vi "RTS Wago Data 1.vi"(8 "Error In":errorcluster, 11 "Chamber 1 Data in":T1 {"Room PID Settings"."Room Dehumid Temperature I (*RM Dehum I1)" max=30000 step=1; "Room PID Settings"."Room Dehumid Temperature P (*RM Dehum P1)" max=30000 step=1; "Room PID Settings"."Room Cool Temperature I (*RM Cool I1)" max=30000 step=1; "Room PID Settings"."Room Cool Temperature P (*RM Cool P1)" max=30000 step=1; "Room PID Settings"."Room Heat I (*RM Heat I1)" max=30000 step=1; "Room PID Settings"."Room Heat P (*RM Heat P1)" max=30000 step=1; "Room PID Settings"."Room Humidity I (*RM Hum I1)" max=30000 step=1; "Room PID Settings"."Room Humidity P (*RM Hum P1)" max=30000 step=1; "Room PID Settings"."Room Dry I (*RM Dry I1)" max=30000 step=1; "Room PID Settings"."Room Dry P(*RM Dry P1)" max=30000 step=1; "Station 8"."Voltage (V):Element 1 Avg" format="%.3g"; "Station 8"."Voltage (V):Element 2 Avg" format="%.3g"; "Station 8"."Max Watt Hours" format="%.3g"; "Station 8"."Power Factor:Element 2" format="%.3g"; "Station 8"."Power Factor:Element 1" format="%.3g"; "Station 8"."Apparent Power (VA):Element 2" format="%.3g"; "Station 8"."Apparent Power (VA):Element 1" format="%.3g"; "Station 8"."Frequency (Hz):Element 1" format="%.3g"; "Station 8"."Time:Element 1" format="%.3g"; "Station 8"."Voltage Crest Factor:Element 2" format="%.3g"; "Station 8"."Voltage Crest Factor:Element 1" format="%.3g"; "Station 8"."Voltage Harmonic (%):Element 2" format="%.3g"; "Station 8"."Voltage Harmonic (%):Element 1" format="%.3g"; "Station 8"."Current Crest Factor:Element 2" format="%.3g"; "Station 8"."Current Crest Factor:Element 1" format="%.3g"; "Station 8"."Voltage (V):Element 1" format="%.3g"; "Station 8"."Voltage (V):Element 2" format="%.3g"; "Station 8"."Watt Hours (Wh):Sigma" format="%.3f"; "Station 8"."Power (W):Sigma" format="%.3g"; "Station 8"."Current (A):Element 2" format="%.3g"; "Station 8"."Current (A):Element 1" format="%.3g"; "Station 7"."Voltage (V):Element 1 Avg" format="%.3g"; "Station 7"."Voltage (V):Element 2 Avg" format="%.3g"; "Station 7"."Max Watt Hours" format="%.3g"; "Station 7"."Power Factor:Element 2" format="%.3g"; "Station 7"."Power Factor:Element 1" format="%.3g"; "Station 7"."Apparent Power (VA):Element 2" format="%.3g"; "Station 7"."Apparent Power (VA):Element 1" format="%.3g"; "Station 7"."Frequency (Hz):Element 1" format="%.3g"; "Station 7"."Time:Element 1" format="%.3g"; "Station 7"."Voltage Crest Factor:Element 2" format="%.3g"; "Station 7"."Voltage Crest Factor:Element 1" format="%.3g"; "Station 7"."Voltage Harmonic (%):Element 2" format="%.3g"; "Station 7"."Voltage Harmonic (%):Element 1" format="%.3g"; "Station 7"."Current Crest Factor:Element 2" format="%.3g"; "Station 7"."Current Crest Factor:Element 1" format="%.3g"; "Station 7"."Voltage (V):Element 1" format="%.3g"; "Station 7"."Voltage (V):Element 2" format="%.3g"; "Station 7"."Watt Hours (Wh):Sigma" format="%.3f"; "Station 7"."Power (W):Sigma" format="%.3g"; "Station 7"."Current (A):Element 2" format="%.3g"; "Station 7"."Current (A):Element 1" format="%.3g"; "Station 6"."Voltage (V):Element 1 Avg" format="%.3g"; "Station 6"."Voltage (V):Element 2 Avg" format="%.3g"; "Station 6"."Max Watt Hours" format="%.3g"; "Station 6"."Power Factor:Element 2" format="%.3g"; "Station 6"."Power Factor:Element 1" format="%.3g"; "Station 6"."Apparent Power (VA):Element 2" format="%.3g"; "Station 6"."Apparent Power (VA):Element 1" format="%.3g"; "Station 6"."Frequency (Hz):Element 1" format="%.3g"; "Station 6"."Time:Element 1" format="%.3g"; "Station 6"."Voltage Crest Factor:Element 2" format="%.3g"; "Station 6"."Voltage Crest Factor:Element 1" format="%.3g"; "Station 6"."Voltage Harmonic (%):Element 2" format="%.3g"; "Station 6"."Voltage Harmonic (%):Element 1" format="%.3g"; "Station 6"."Current Crest Factor:Element 2" format="%.3g"; "Station 6"."Current Crest Factor:Element 1" format="%.3g"; "Station 6"."Voltage (V):Element 1" format="%.3g"; "Station 6"."Voltage (V):Element 2" format="%.3g"; "Station 6"."Watt Hours (Wh):Sigma" format="%.3f"; "Station 6"."Power (W):Sigma" format="%.3g"; "Station 6"."Current (A):Element 2" format="%.3g"; "Station 6"."Current (A):Element 1" format="%.3g"; "Station 5"."Voltage (V):Element 1 Avg" format="%.3g"; "Station 5"."Voltage (V):Element 2 Avg" format="%.3g"; "Station 5"."Max Watt Hours" format="%.3g"; "Station 5"."Power Factor:Element 2" format="%.3g"; "Station 5"."Power Factor:Element 1" format="%.3g"; "Station 5"."Apparent Power (VA):Element 2" format="%.3g"; "Station 5"."Apparent Power (VA):Element 1" format="%.3g"; "Station 5"."Frequency (Hz):Element 1" format="%.3g"; "Station 5"."Time:Element 1" format="%.3g"; "Station 5"."Voltage Crest Factor:Element 2" format="%.3g"; "Station 5"."Voltage Crest Factor:Element 1" format="%.3g"; "Station 5"."Voltage Harmonic (%):Element 2" format="%.3g"; "Station 5"."Voltage Harmonic (%):Element 1" format="%.3g"; "Station 5"."Current Crest Factor:Element 2" format="%.3g"; "Station 5"."Current Crest Factor:Element 1" format="%.3g"; "Station 5"."Voltage (V):Element 1" format="%.3g"; "Station 5"."Voltage (V):Element 2" format="%.3g"; "Station 5"."Watt Hours (Wh):Sigma" format="%.3f"; "Station 5"."Power (W):Sigma" format="%.3g"; "Station 5"."Current (A):Element 2" format="%.3g"; "Station 5"."Current (A):Element 1" format="%.3g"; "Station 4"."Voltage (V):Element 1 Avg" format="%.3g"; "Station 4"."Voltage (V):Element 2 Avg" format="%.3g"; "Station 4"."Max Watt Hours" format="%.3g"; "Station 4"."Power Factor:Element 2" format="%.3g"; "Station 4"."Power Factor:Element 1" format="%.3g"; "Station 4"."Apparent Power (VA):Element 2" format="%.3g"; "Station 4"."Apparent Power (VA):Element 1" format="%.3g"; "Station 4"."Frequency (Hz):Element 1" format="%.3g"; "Station 4"."Time:Element 1" format="%.3g"; "Station 4"."Voltage Crest Factor:Element 2" format="%.3g"; "Station 4"."Voltage Crest Factor:Element 1" format="%.3g"; "Station 4"."Voltage Harmonic (%):Element 2" format="%.3g"; "Station 4"."Voltage Harmonic (%):Element 1" format="%.3g"; "Station 4"."Current Crest Factor:Element 2" format="%.3g"; "Station 4"."Current Crest Factor:Element 1" format="%.3g"; "Station 4"."Voltage (V):Element 1" format="%.3g"; "Station 4"."Voltage (V):Element 2" format="%.3g"; "Station 4"."Watt Hours (Wh):Sigma" format="%.3f"; "Station 4"."Power (W):Sigma" format="%.3g"; "Station 4"."Current (A):Element 2" format="%.3g"; "Station 4"."Current (A):Element 1" format="%.3g"; "Station 3"."Voltage (V):Element 1 Avg" format="%.3g"; "Station 3"."Voltage (V):Element 2 Avg" format="%.3g"; "Station 3"."Max Watt Hours" format="%.3g"; "Station 3"."Power Factor:Element 2" format="%.3g"; "Station 3"."Power Factor:Element 1" format="%.3g"; "Station 3"."Apparent Power (VA):Element 2" format="%.3g"; "Station 3"."Apparent Power (VA):Element 1" format="%.3g"; "Station 3"."Frequency (Hz):Element 1" format="%.3g"; "Station 3"."Time:Element 1" format="%.3g"; "Station 3"."Voltage Crest Factor:Element 2" format="%.3g"; "Station 3"."Voltage Crest Factor:Element 1" format="%.3g"; "Station 3"."Voltage Harmonic (%):Element 2" format="%.3g"; "Station 3"."Voltage Harmonic (%):Element 1" format="%.3g"; "Station 3"."Current Crest Factor:Element 2" format="%.3g"; "Station 3"."Current Crest Factor:Element 1" format="%.3g"; "Station 3"."Voltage (V):Element 1" format="%.3g"; "Station 3"."Voltage (V):Element 2" format="%.3g"; "Station 3"."Watt Hours (Wh):Sigma" format="%.3f"; "Station 3"."Power (W):Sigma" format="%.3g"; "Station 3"."Current (A):Element 2" format="%.3g"; "Station 3"."Current (A):Element 1" format="%.3g"; "Station 2"."Voltage (V):Element 1 Avg" format="%.3g"; "Station 2"."Voltage (V):Element 2 Avg" format="%.3g"; "Station 2"."Max Watt Hours" format="%.3g"; "Station 2"."Power Factor:Element 2" format="%.3g"; "Station 2"."Power Factor:Element 1" format="%.3g"; "Station 2"."Apparent Power (VA):Element 2" format="%.3g"; "Station 2"."Apparent Power (VA):Element 1" format="%.3g"; "Station 2"."Frequency (Hz):Element 1" format="%.3g"; "Station 2"."Time:Element 1" format="%.3g"; "Station 2"."Voltage Crest Factor:Element 2" format="%.3g"; "Station 2"."Voltage Crest Factor:Element 1" format="%.3g"; "Station 2"."Voltage Harmonic (%):Element 2" format="%.3g"; "Station 2"."Voltage Harmonic (%):Element 1" format="%.3g"; "Station 2"."Current Crest Factor:Element 2" format="%.3g"; "Station 2"."Current Crest Factor:Element 1" format="%.3g"; "Station 2"."Voltage (V):Element 1" format="%.3g"; "Station 2"."Voltage (V):Element 2" format="%.3g"; "Station 2"."Watt Hours (Wh):Sigma" format="%.3f"; "Station 2"."Power (W):Sigma" format="%.3g"; "Station 2"."Current (A):Element 2" format="%.3g"; "Station 2"."Current (A):Element 1" format="%.3g"; "Station 1"."Voltage (V):Element 1 Avg" format="%.3g"; "Station 1"."Voltage (V):Element 2 Avg" format="%.3g"; "Station 1"."Max Watt Hours" format="%.3g"; "Station 1"."Power Factor:Element 2" format="%.3g"; "Station 1"."Power Factor:Element 1" format="%.3g"; "Station 1"."Apparent Power (VA):Element 2" format="%.3g"; "Station 1"."Apparent Power (VA):Element 1" format="%.3g"; "Station 1"."Frequency (Hz):Element 1" format="%.3g"; "Station 1"."Time:Element 1" format="%.3g"; "Station 1"."Voltage Crest Factor:Element 2" format="%.3g"; "Station 1"."Voltage Crest Factor:Element 1" format="%.3g"; "Station 1"."Voltage Harmonic (%):Element 2" format="%.3g"; "Station 1"."Voltage Harmonic (%):Element 1" format="%.3g"; "Station 1"."Current Crest Factor:Element 2" format="%.3g"; "Station 1"."Current Crest Factor:Element 1" format="%.3g"; "Station 1"."Voltage (V):Element 1" format="%.3g"; "Station 1"."Voltage (V):Element 2" format="%.3g"; "Station 1"."Watt Hours (Wh):Sigma" format="%.3f"; "Station 1"."Power (W):Sigma" format="%.3g"; "Station 1"."Current (A):Element 2" format="%.3g"; "Station 1"."Current (A):Element 1" format="%.3g"}) -> (0 "Error Out":errorcluster, 1 "Data (DBL)":dbl[](array[numeric]), 2 "Data 1 Output":string[][](array[string]), 3 "Chamber 1 Data Out":T1 {"Room PID Settings"."Room Dehumid Temperature I (*RM Dehum I1)" max=30000 step=1; "Room PID Settings"."Room Dehumid Temperature P (*RM Dehum P1)" max=30000 step=1; "Room PID Settings"."Room Cool Temperature I (*RM Cool I1)" max=30000 step=1; "Room PID Settings"."Room Cool Temperature P (*RM Cool P1)" max=30000 step=1; "Room PID Settings"."Room Heat I (*RM Heat I1)" max=30000 step=1; "Room PID Settings"."Room Heat P (*RM Heat P1)" max=30000 step=1; "Room PID Settings"."Room Humidity I (*RM Hum I1)" max=30000 step=1; "Room PID Settings"."Room Humidity P (*RM Hum P1)" max=30000 step=1; "Room PID Settings"."Room Dry I (*RM Dry I1)" max=30000 step=1; "Room PID Settings"."Room Dry P(*RM Dry P1)" max=30000 step=1; "Station 8"."Voltage (V):Element 1 Avg" format="%.3g"; "Station 8"."Voltage (V):Element 2 Avg" format="%.3g"; "Station 8"."Max Watt Hours" format="%.3g"; "Station 8"."Power Factor:Element 2" format="%.3g"; "Station 8"."Power Factor:Element 1" format="%.3g"; "Station 8"."Apparent Power (VA):Element 2" format="%.3g"; "Station 8"."Apparent Power (VA):Element 1" format="%.3g"; "Station 8"."Frequency (Hz):Element 1" format="%.3g"; "Station 8"."Time:Element 1" format="%.3g"; "Station 8"."Voltage Crest Factor:Element 2" format="%.3g"; "Station 8"."Voltage Crest Factor:Element 1" format="%.3g"; "Station 8"."Voltage Harmonic (%):Element 2" format="%.3g"; "Station 8"."Voltage Harmonic (%):Element 1" format="%.3g"; "Station 8"."Current Crest Factor:Element 2" format="%.3g"; "Station 8"."Current Crest Factor:Element 1" format="%.3g"; "Station 8"."Voltage (V):Element 1" format="%.3g"; "Station 8"."Voltage (V):Element 2" format="%.3g"; "Station 8"."Watt Hours (Wh):Sigma" format="%.3f"; "Station 8"."Power (W):Sigma" format="%.3g"; "Station 8"."Current (A):Element 2" format="%.3g"; "Station 8"."Current (A):Element 1" format="%.3g"; "Station 7"."Voltage (V):Element 1 Avg" format="%.3g"; "Station 7"."Voltage (V):Element 2 Avg" format="%.3g"; "Station 7"."Max Watt Hours" format="%.3g"; "Station 7"."Power Factor:Element 2" format="%.3g"; "Station 7"."Power Factor:Element 1" format="%.3g"; "Station 7"."Apparent Power (VA):Element 2" format="%.3g"; "Station 7"."Apparent Power (VA):Element 1" format="%.3g"; "Station 7"."Frequency (Hz):Element 1" format="%.3g"; "Station 7"."Time:Element 1" format="%.3g"; "Station 7"."Voltage Crest Factor:Element 2" format="%.3g"; "Station 7"."Voltage Crest Factor:Element 1" format="%.3g"; "Station 7"."Voltage Harmonic (%):Element 2" format="%.3g"; "Station 7"."Voltage Harmonic (%):Element 1" format="%.3g"; "Station 7"."Current Crest Factor:Element 2" format="%.3g"; "Station 7"."Current Crest Factor:Element 1" format="%.3g"; "Station 7"."Voltage (V):Element 1" format="%.3g"; "Station 7"."Voltage (V):Element 2" format="%.3g"; "Station 7"."Watt Hours (Wh):Sigma" format="%.3f"; "Station 7"."Power (W):Sigma" format="%.3g"; "Station 7"."Current (A):Element 2" format="%.3g"; "Station 7"."Current (A):Element 1" format="%.3g"; "Station 6"."Voltage (V):Element 1 Avg" format="%.3g"; "Station 6"."Voltage (V):Element 2 Avg" format="%.3g"; "Station 6"."Max Watt Hours" format="%.3g"; "Station 6"."Power Factor:Element 2" format="%.3g"; "Station 6"."Power Factor:Element 1" format="%.3g"; "Station 6"."Apparent Power (VA):Element 2" format="%.3g"; "Station 6"."Apparent Power (VA):Element 1" format="%.3g"; "Station 6"."Frequency (Hz):Element 1" format="%.3g"; "Station 6"."Time:Element 1" format="%.3g"; "Station 6"."Voltage Crest Factor:Element 2" format="%.3g"; "Station 6"."Voltage Crest Factor:Element 1" format="%.3g"; "Station 6"."Voltage Harmonic (%):Element 2" format="%.3g"; "Station 6"."Voltage Harmonic (%):Element 1" format="%.3g"; "Station 6"."Current Crest Factor:Element 2" format="%.3g"; "Station 6"."Current Crest Factor:Element 1" format="%.3g"; "Station 6"."Voltage (V):Element 1" format="%.3g"; "Station 6"."Voltage (V):Element 2" format="%.3g"; "Station 6"."Watt Hours (Wh):Sigma" format="%.3f"; "Station 6"."Power (W):Sigma" format="%.3g"; "Station 6"."Current (A):Element 2" format="%.3g"; "Station 6"."Current (A):Element 1" format="%.3g"; "Station 5"."Voltage (V):Element 1 Avg" format="%.3g"; "Station 5"."Voltage (V):Element 2 Avg" format="%.3g"; "Station 5"."Max Watt Hours" format="%.3g"; "Station 5"."Power Factor:Element 2" format="%.3g"; "Station 5"."Power Factor:Element 1" format="%.3g"; "Station 5"."Apparent Power (VA):Element 2" format="%.3g"; "Station 5"."Apparent Power (VA):Element 1" format="%.3g"; "Station 5"."Frequency (Hz):Element 1" format="%.3g"; "Station 5"."Time:Element 1" format="%.3g"; "Station 5"."Voltage Crest Factor:Element 2" format="%.3g"; "Station 5"."Voltage Crest Factor:Element 1" format="%.3g"; "Station 5"."Voltage Harmonic (%):Element 2" format="%.3g"; "Station 5"."Voltage Harmonic (%):Element 1" format="%.3g"; "Station 5"."Current Crest Factor:Element 2" format="%.3g"; "Station 5"."Current Crest Factor:Element 1" format="%.3g"; "Station 5"."Voltage (V):Element 1" format="%.3g"; "Station 5"."Voltage (V):Element 2" format="%.3g"; "Station 5"."Watt Hours (Wh):Sigma" format="%.3f"; "Station 5"."Power (W):Sigma" format="%.3g"; "Station 5"."Current (A):Element 2" format="%.3g"; "Station 5"."Current (A):Element 1" format="%.3g"; "Station 4"."Voltage (V):Element 1 Avg" format="%.3g"; "Station 4"."Voltage (V):Element 2 Avg" format="%.3g"; "Station 4"."Max Watt Hours" format="%.3g"; "Station 4"."Power Factor:Element 2" format="%.3g"; "Station 4"."Power Factor:Element 1" format="%.3g"; "Station 4"."Apparent Power (VA):Element 2" format="%.3g"; "Station 4"."Apparent Power (VA):Element 1" format="%.3g"; "Station 4"."Frequency (Hz):Element 1" format="%.3g"; "Station 4"."Time:Element 1" format="%.3g"; "Station 4"."Voltage Crest Factor:Element 2" format="%.3g"; "Station 4"."Voltage Crest Factor:Element 1" format="%.3g"; "Station 4"."Voltage Harmonic (%):Element 2" format="%.3g"; "Station 4"."Voltage Harmonic (%):Element 1" format="%.3g"; "Station 4"."Current Crest Factor:Element 2" format="%.3g"; "Station 4"."Current Crest Factor:Element 1" format="%.3g"; "Station 4"."Voltage (V):Element 1" format="%.3g"; "Station 4"."Voltage (V):Element 2" format="%.3g"; "Station 4"."Watt Hours (Wh):Sigma" format="%.3f"; "Station 4"."Power (W):Sigma" format="%.3g"; "Station 4"."Current (A):Element 2" format="%.3g"; "Station 4"."Current (A):Element 1" format="%.3g"; "Station 3"."Voltage (V):Element 1 Avg" format="%.3g"; "Station 3"."Voltage (V):Element 2 Avg" format="%.3g"; "Station 3"."Max Watt Hours" format="%.3g"; "Station 3"."Power Factor:Element 2" format="%.3g"; "Station 3"."Power Factor:Element 1" format="%.3g"; "Station 3"."Apparent Power (VA):Element 2" format="%.3g"; "Station 3"."Apparent Power (VA):Element 1" format="%.3g"; "Station 3"."Frequency (Hz):Element 1" format="%.3g"; "Station 3"."Time:Element 1" format="%.3g"; "Station 3"."Voltage Crest Factor:Element 2" format="%.3g"; "Station 3"."Voltage Crest Factor:Element 1" format="%.3g"; "Station 3"."Voltage Harmonic (%):Element 2" format="%.3g"; "Station 3"."Voltage Harmonic (%):Element 1" format="%.3g"; "Station 3"."Current Crest Factor:Element 2" format="%.3g"; "Station 3"."Current Crest Factor:Element 1" format="%.3g"; "Station 3"."Voltage (V):Element 1" format="%.3g"; "Station 3"."Voltage (V):Element 2" format="%.3g"; "Station 3"."Watt Hours (Wh):Sigma" format="%.3f"; "Station 3"."Power (W):Sigma" format="%.3g"; "Station 3"."Current (A):Element 2" format="%.3g"; "Station 3"."Current (A):Element 1" format="%.3g"; "Station 2"."Voltage (V):Element 1 Avg" format="%.3g"; "Station 2"."Voltage (V):Element 2 Avg" format="%.3g"; "Station 2"."Max Watt Hours" format="%.3g"; "Station 2"."Power Factor:Element 2" format="%.3g"; "Station 2"."Power Factor:Element 1" format="%.3g"; "Station 2"."Apparent Power (VA):Element 2" format="%.3g"; "Station 2"."Apparent Power (VA):Element 1" format="%.3g"; "Station 2"."Frequency (Hz):Element 1" format="%.3g"; "Station 2"."Time:Element 1" format="%.3g"; "Station 2"."Voltage Crest Factor:Element 2" format="%.3g"; "Station 2"."Voltage Crest Factor:Element 1" format="%.3g"; "Station 2"."Voltage Harmonic (%):Element 2" format="%.3g"; "Station 2"."Voltage Harmonic (%):Element 1" format="%.3g"; "Station 2"."Current Crest Factor:Element 2" format="%.3g"; "Station 2"."Current Crest Factor:Element 1" format="%.3g"; "Station 2"."Voltage (V):Element 1" format="%.3g"; "Station 2"."Voltage (V):Element 2" format="%.3g"; "Station 2"."Watt Hours (Wh):Sigma" format="%.3f"; "Station 2"."Power (W):Sigma" format="%.3g"; "Station 2"."Current (A):Element 2" format="%.3g"; "Station 2"."Current (A):Element 1" format="%.3g"; "Station 1"."Voltage (V):Element 1 Avg" format="%.3g"; "Station 1"."Voltage (V):Element 2 Avg" format="%.3g"; "Station 1"."Max Watt Hours" format="%.3g"; "Station 1"."Power Factor:Element 2" format="%.3g"; "Station 1"."Power Factor:Element 1" format="%.3g"; "Station 1"."Apparent Power (VA):Element 2" format="%.3g"; "Station 1"."Apparent Power (VA):Element 1" format="%.3g"; "Station 1"."Frequency (Hz):Element 1" format="%.3g"; "Station 1"."Time:Element 1" format="%.3g"; "Station 1"."Voltage Crest Factor:Element 2" format="%.3g"; "Station 1"."Voltage Crest Factor:Element 1" format="%.3g"; "Station 1"."Voltage Harmonic (%):Element 2" format="%.3g"; "Station 1"."Voltage Harmonic (%):Element 1" format="%.3g"; "Station 1"."Current Crest Factor:Element 2" format="%.3g"; "Station 1"."Current Crest Factor:Element 1" format="%.3g"; "Station 1"."Voltage (V):Element 1" format="%.3g"; "Station 1"."Voltage (V):Element 2" format="%.3g"; "Station 1"."Watt Hours (Wh):Sigma" format="%.3f"; "Station 1"."Power (W):Sigma" format="%.3g"; "Station 1"."Current (A):Element 2" format="%.3g"; "Station 1"."Current (A):Element 1" format="%.3g"})   [LabVIEW 2016]
uses:
  Type Definitions/RTS Chamber Data.ctl
  Utility/Type Definitions/UTILITY Power Data.ctl
  Type Definitions/RTS Chamber TCs.ctl
  Type Definitions/RTS MX5 AUX Data.ctl
  Drivers/WAGO 750-881/Type Definitions/Wago Door Relays.ctl
  Drivers/WAGO 750-881/Type Definitions/Wago Contactor Settings.ctl
  Drivers/WAGO 750-881/Type Definitions/Wago Ground Leakage.ctl
  Drivers/WAGO 750-881/Type Definitions/Wago Measured Input Data.ctl
  Drivers/WAGO 750-881/Type Definitions/Wago Room Setpoint Targets.ctl
  Drivers/WAGO 750-881/Type Definitions/Wago Room PID Settings.ctl
  Drivers/WAGO 750-881/Type Definitions/Wago Room Condtions.ctl
panel:
  # "APLUS"
  # "MX100"
  # "Wago Controller"
  # "APLUS"
  # "MX100"
  # "Wago Controller"
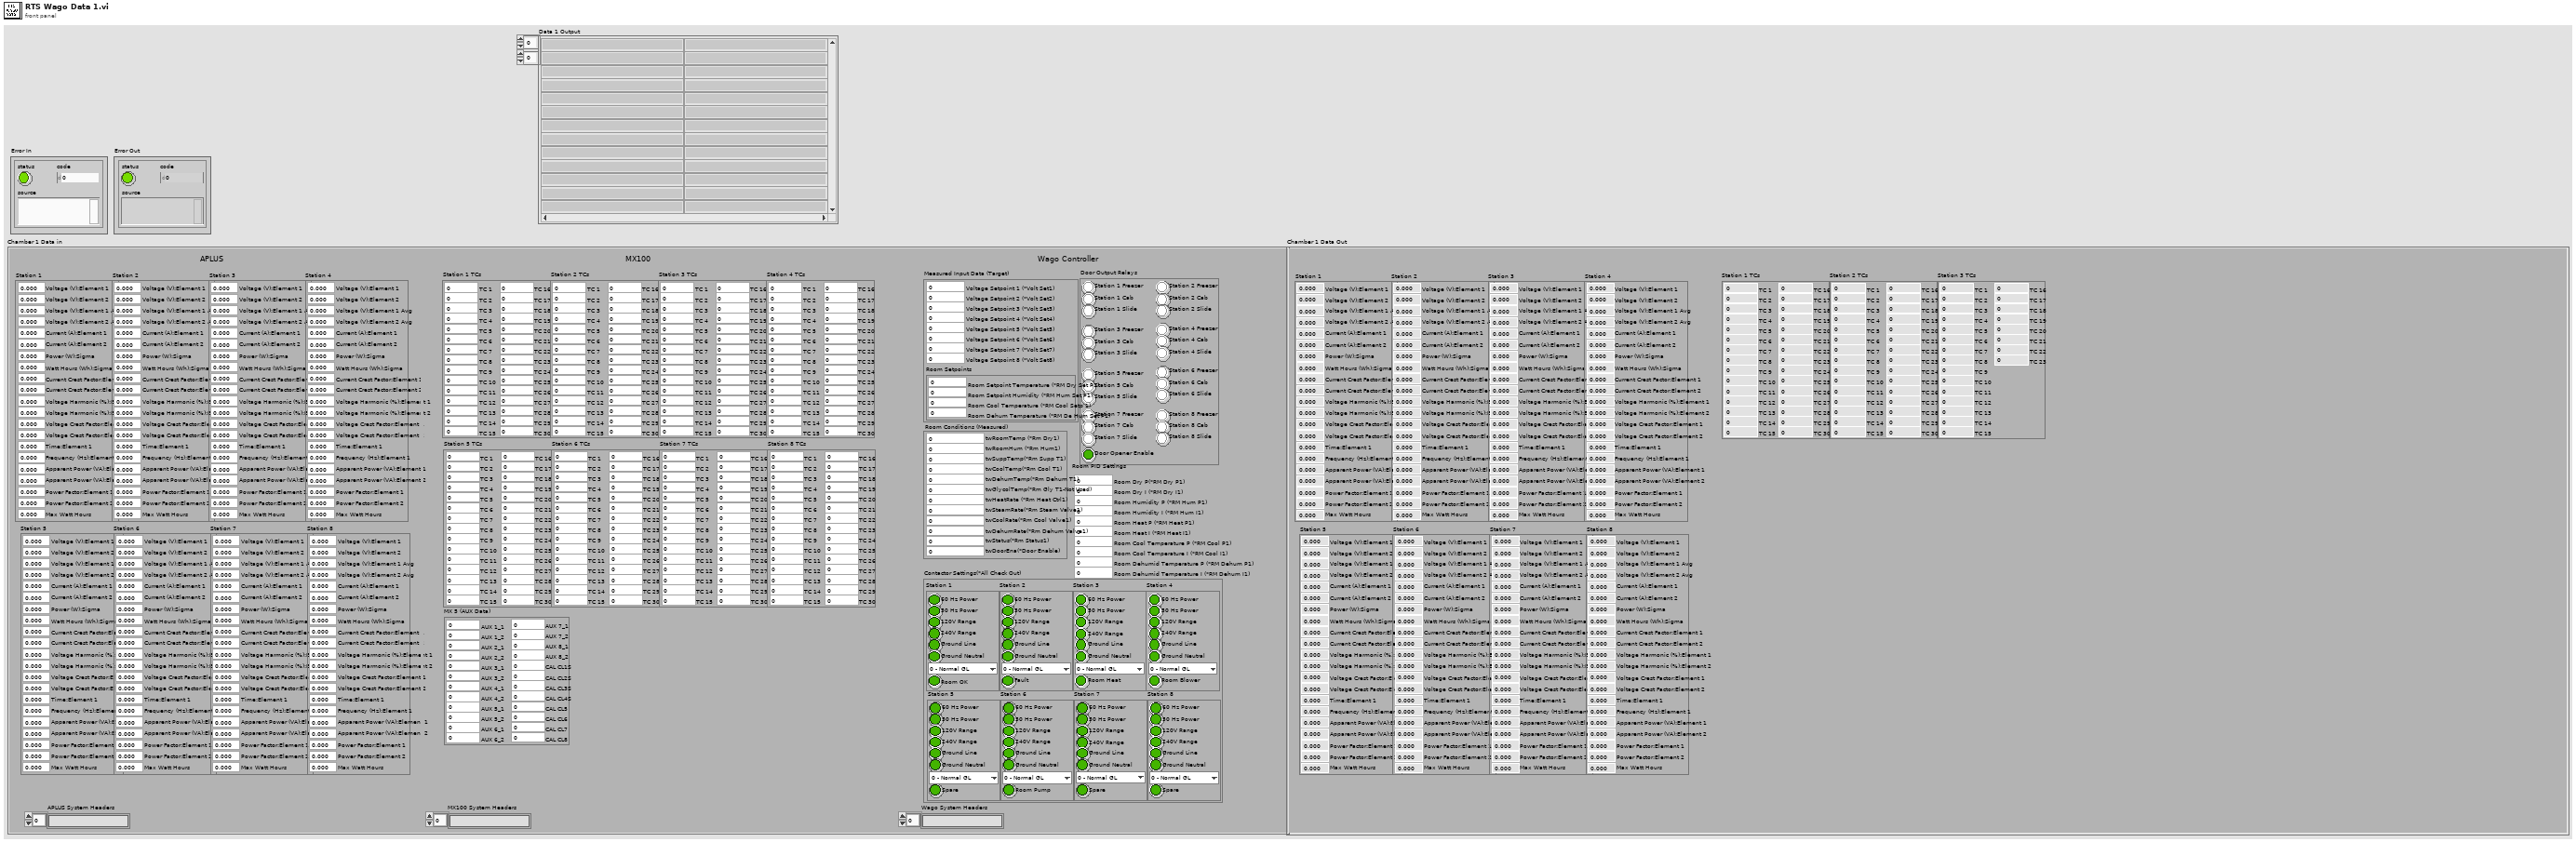
[diagram p1: front panel]
types:
  T1 = typedef "RTS Chamber Data.ctl" = cluster{"Station 1":T2, "Station 2":T2, "Station 3":T2, "Station 4":T2, "Station 5":T2, "Station 6":T2, "Station 7":T2, "Station 8":T2, "Station 1 TCs":T3, "Station 2 TCs":T3, "Station 3 TCs":T3, "Station 4 TCs":T3, "Station 5 TCs":T3, "Station 6 TCs":T3, "Station 7 TCs":T3, "Station 8 TCs":T3, "MX 5 (AUX Data)":T4, "Door Output Relays":T5, "Contactor Settings(*All Check Out)":T6, "Measured Input Data (Target)":T8, "Room PID Settings":T10, "Room Conditions (Measured)":T11, "APLUS System Headers":string[], "MX100 System Headers":string[], "Wago System Headers":string[]}
  T2 = typedef "UTILITY Power Data.ctl" = cluster{"Current (A):Element 1":dbl, "Current (A):Element 2":dbl, "Power (W):Sigma":dbl, "Watt Hours (Wh):Sigma":dbl, "Voltage (V):Element 2":dbl, "Voltage (V):Element 1":dbl, "Current Crest Factor:Element 1":dbl, "Current Crest Factor:Element 2":dbl, "Voltage Harmonic (%):Element 1":dbl, "Voltage Harmonic (%):Element 2":dbl, "Voltage Crest Factor:Element 1":dbl, "Voltage Crest Factor:Element 2":dbl, "Time:Element 1":dbl, "Frequency (Hz):Element 1":dbl, "Apparent Power (VA):Element 1":dbl, "Apparent Power (VA):Element 2":dbl, "Power Factor:Element 1":dbl, "Power Factor:Element 2":dbl, "Max Watt Hours":dbl, "Voltage (V):Element 2 Avg":dbl, "Voltage (V):Element 1 Avg":dbl}
  T3 = typedef "RTS Chamber TCs.ctl" = cluster{"TC 1":dbl, "TC 2":dbl, "TC 3":dbl, "TC 4":dbl, "TC 5":dbl, "TC 6":dbl, "TC 7":dbl, "TC 8":dbl, "TC 9":dbl, "TC 10":dbl, "TC 11":dbl, "TC 12":dbl, "TC 13":dbl, "TC 14":dbl, "TC 15":dbl, "TC 16":dbl, "TC 17":dbl, "TC 18":dbl, "TC 19":dbl, "TC 20":dbl, "TC 21":dbl, "TC 22":dbl, "TC 23":dbl, "TC 24":dbl, "TC 25":dbl, "TC 26":dbl, "TC 27":dbl, "TC 28":dbl, "TC 29":dbl, "TC 30":dbl}
  T4 = typedef "RTS MX5 AUX Data.ctl" = cluster{"AUX 1_1":dbl, "AUX 1_2":dbl, "AUX 2_1":dbl, "AUX 2_2":dbl, "AUX 3_1":dbl, "AUX 3_2":dbl, "AUX 4_1":dbl, "AUX 4_2":dbl, "AUX 5_1":dbl, "AUX 5_2":dbl, "AUX 6_1":dbl, "AUX 6_2":dbl, "AUX 7_1":dbl, "AUX 7_2":dbl, "AUX 8_1":dbl, "AUX 8_2":dbl, "CAL CL1S":dbl, "CAL CL2S":dbl, "CAL CL3S":dbl, "CAL CL4S":dbl, "CAL CL5":dbl, "CAL CL6":dbl, "CAL CL7":dbl, "CAL CL8":dbl}
  T5 = typedef "Wago Door Relays.ctl" = cluster{"Station 1 Freezer":bool, "Station 1 Cab":bool, "Station 1 Slide":bool, "Station 2 Freezer":bool, "Station 2 Cab":bool, "Station 2 Slide":bool, "Station 3 Freezer":bool, "Station 3 Cab":bool, "Station 3 Slide":bool, "Station 4 Freezer":bool, "Station 4 Cab":bool, "Station 4 Slide":bool, "Station 5 Freezer":bool, "Station 5 Cab":bool, "Station 5 Slide":bool, "Station 6 Freezer":bool, "Station 6 Cab":bool, "Station 6 Slide":bool, "Station 7 Freezer":bool, "Station 7 Cab":bool, "Station 7 Slide":bool, "Station 8 Freezer":bool, "Station 8 Cab":bool, "Station 8 Slide":bool, "Door Opener Enable":bool}
  T6 = typedef "Wago Contactor Settings.ctl" = cluster{"Station 1":cluster{"60 Hz Power":bool, "50 Hz Power":bool, "120V Range":bool, "240V Range":bool, "Ground Line":bool, "Ground Neutral":bool, "Room OK":bool, "Ground Leakage":T7}, "Station 2":cluster{"60 Hz Power":bool, "50 Hz Power":bool, "120V Range":bool, "240V Range":bool, "Ground Line":bool, "Ground Neutral":bool, "Fault":bool, "Ground Leakage":T7}, "Station 3":cluster{"60 Hz Power":bool, "50 Hz Power":bool, "120V Range":bool, "240V Range":bool, "Ground Line":bool, "Ground Neutral":bool, "Room Heat":bool, "Ground Leakage":T7}, "Station 4":cluster{"60 Hz Power":bool, "50 Hz Power":bool, "120V Range":bool, "240V Range":bool, "Ground Line":bool, "Ground Neutral":bool, "Room Blower":bool, "Ground Leakage":T7}, "Station 5":cluster{"60 Hz Power":bool, "50 Hz Power":bool, "120V Range":bool, "240V Range":bool, "Ground Line":bool, "Ground Neutral":bool, "Spare":bool, "Ground Leakage":T7}, "Station 6":cluster{"60 Hz Power":bool, "50 Hz Power":bool, "120V Range":bool, "240V Range":bool, "Ground Line":bool, "Ground Neutral":bool, "Room Pump":bool, "Ground Leakage":T7}, "Station 7":cluster{"60 Hz Power":bool, "50 Hz Power":bool, "120V Range":bool, "240V Range":bool, "Ground Line":bool, "Ground Neutral":bool, "Spare":bool, "Ground Leakage":T7}, "Station 8":cluster{"60 Hz Power":bool, "50 Hz Power":bool, "120V Range":bool, "240V Range":bool, "Ground Line":bool, "Ground Neutral":bool, "Spare":bool, "Ground Leakage":T7}}
  T7 = typedef "Wago Ground Leakage.ctl" = enum16{"0 - Normal GL", "1 - Measure GL"}
  T8 = typedef "Wago Measured Input Data.ctl" = cluster{"Voltage Setpoint 1 (*Volt Set1)":dbl, "Voltage Setpoint 2 (*Volt Set2)":dbl, "Voltage Setpoint 3 (*Volt Set3)":dbl, "Voltage Setpoint 4 (*Volt Set4)":dbl, "Voltage Setpoint 5 (*Volt Set5)":dbl, "Voltage Setpoint 6 (*Volt Set6)":dbl, "Voltage Setpoint 7 (*Volt Set7)":dbl, "Voltage Setpoint 8 (*Volt Set8)":dbl, "Room Setpoints":T9}
  T9 = typedef "Wago Room Setpoint Targets.ctl" = cluster{"Room Setpoint Temperature (*RM Dry Set P1)":dbl, "Room Setpoint Humidity (*RM Hum Set P1)":dbl, "Room Cool Temperature (*RM Cool Setp 1)":dbl, "Room Dehum Temperature (*RM De Hum Set P1)":dbl}
  T10 = typedef "Wago Room PID Settings.ctl" = cluster{"Room Dry P(*RM Dry P1)":u16, "Room Dry I (*RM Dry I1)":u16, "Room Humidity P (*RM Hum P1)":u16, "Room Humidity I (*RM Hum I1)":u16, "Room Heat P (*RM Heat P1)":u16, "Room Heat I (*RM Heat I1)":u16, "Room Cool Temperature P (*RM Cool P1)":u16, "Room Cool Temperature I (*RM Cool I1)":u16, "Room Dehumid Temperature P (*RM Dehum P1)":u16, "Room Dehumid Temperature I (*RM Dehum I1)":u16}
  T11 = typedef "Wago Room Condtions.ctl" = cluster{"twDoorEna(*Door Enable)":u16, "twStatus(*Rm Status1)":u16, "twRoomTemp (*Rm Dry1)":dbl, "twRoomHum (*Rm Hum1)":dbl, "twSuppTemp(*Rm Supp T1)":dbl, "twCoolTemp(*Rm Cool T1)":dbl, "twDehumTemp(*Rm Dehum T1)":dbl, "twGlycolTemp(*Rm Gly T1-Not Used)":dbl, "twDehumRate(*Rm Dehum Valve1)":dbl, "twCoolRate(*Rm Cool Valve1)":dbl, "twSteamRate(*Rm Steam Valve1)":dbl, "twHeatRate (*Rm Heat Ctrl1)":dbl}
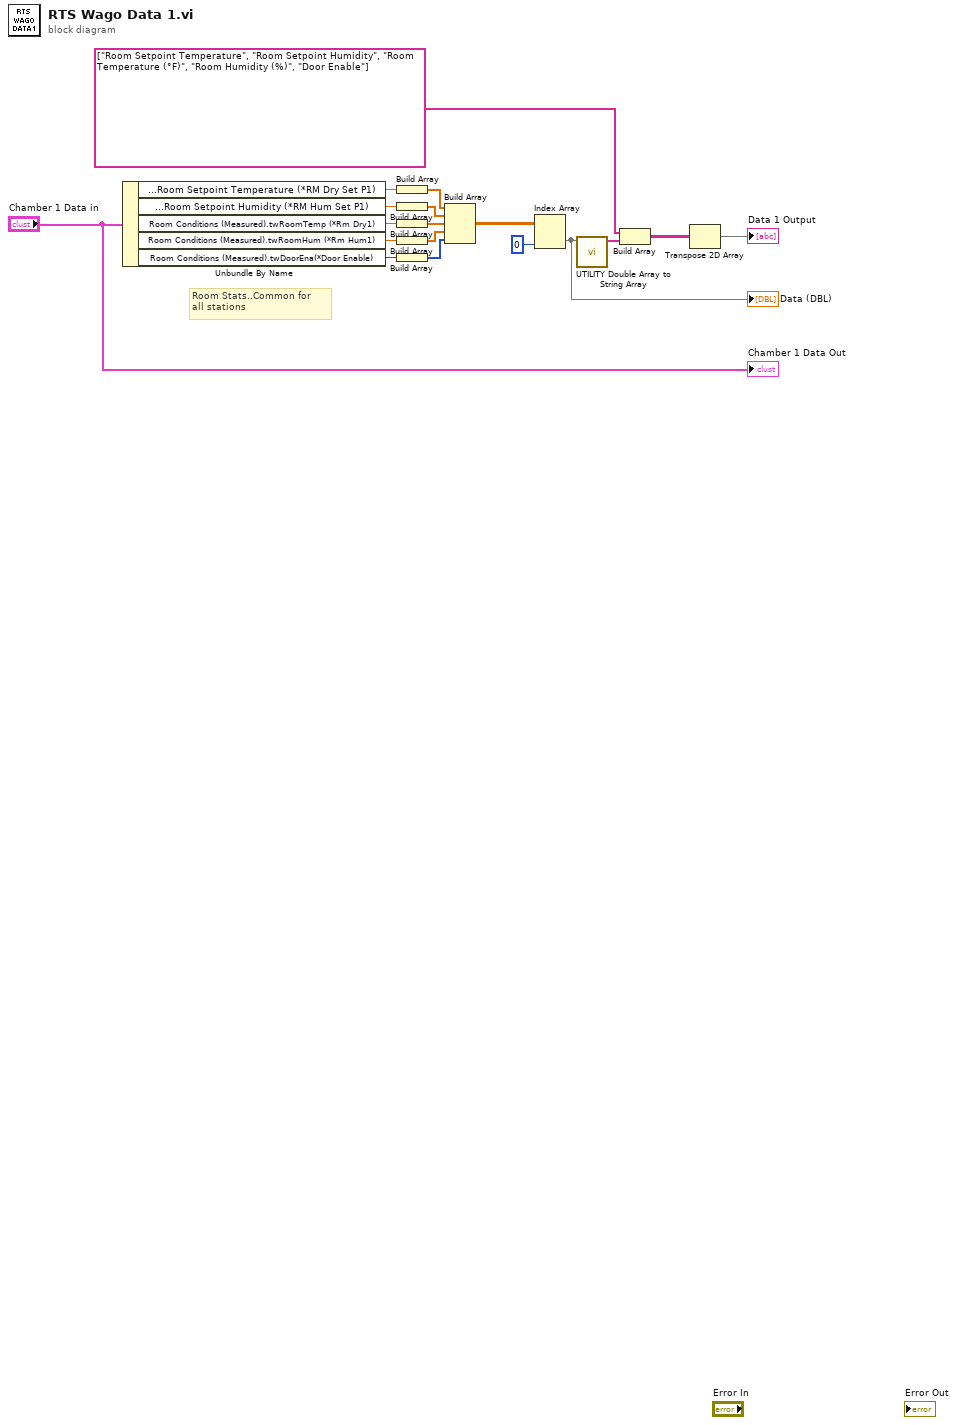
[diagram p0: block diagram]
diagram:
  # "Room Stats..Common for \nall stations"
  n1 = Unbundle By Name("Chamber 1 Data in") -> ("Measured Input Data (Target).Room Setpoints.Room Setpoint Temperature (*RM Dry Set P1)"=w3:dbl, "Measured Input Data (Target).Room Setpoints.Room Setpoint Humidity (*RM Hum Set P1)"=w4:dbl, "Room Conditions (Measured).twRoomTemp (*Rm Dry1)"=w5:dbl, "Room Conditions (Measured).twRoomHum (*Rm Hum1)"=w6:dbl, "Room Conditions (Measured).twDoorEna(*Door Enable)"=w7:u16)
  n2 = Build Array(w3) -> (w13:dbl[])
  n3 = Build Array(w4) -> (w14:dbl[])
  n4 = Build Array(w5) -> (w15:dbl[])
  n5 = Build Array(w6) -> (w16:dbl[])
  n6 = Build Array(w7) -> (w17:u16[])
  n7 = Build Array(w13, w14, w15, w16, w17) -> (w11:dbl[][])
  n8 = Index Array(array=w11, index (col)=0 ("disabled index (col)")) -> (element=w9:dbl[])  [unwired: 1 in]
  "Data (DBL)" <- w9
  n9 = call "UTILITY Double Array to String Array.vi"("Hex Array Out"=w9) -> ("Array"=w12:string[])  [unwired: 10 in]
  n10 = Build Array(string[] ["Room Setpoint Temperature", "Room Setpoint Humidity", "Room Temperature (°F)", "Room Humidity (%)", "Door Enable"], w12) -> (w2:string[][])
  n11 = Transpose 2D Array(2D array=w2) -> (transposed array=→"Data 1 Output":string[][])
  "Chamber 1 Data Out" <- "Chamber 1 Data in"
